vi "SetupApplication.vi"(8 "error in (no error)":errorcluster) -> (0 "error out":errorcluster)   [LabVIEW 2011]
uses:
  080 - TOOLS/Traduction/Dictionnary/EnumCommandDictionnaire.ctl
  050 - CONFIG/00 - ApplicationConfig/Ctrls/EnumFgvConfigCommand.ctl
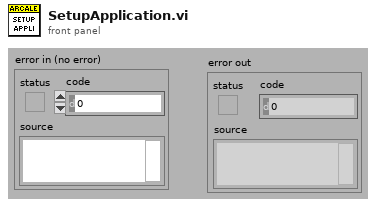
[diagram p1: front panel]
types:
  T1 = typedef "EnumCommandDictionnaire.ctl" = enum16{"Load", "Translate", "Save", "GetDico", "Set : A traduire = Vrai", "Set : A Traduire = Faux", "SetDico"}
  T2 = typedef "EnumFgvConfigCommand.ctl" = enum16{"Load", "Get", "Set", "Save To Disk"}
  T3 = typedef "ApplicationConfig.ctl" = cluster{"Data Path":path, "MessageHandlerConfig":T4, "Simulation":bool, "Dictionnary":string}
  T4 = typedef "MessageHandlerConfig.ctl" = cluster{"Max log files":u32, "Max messages per file":u32}
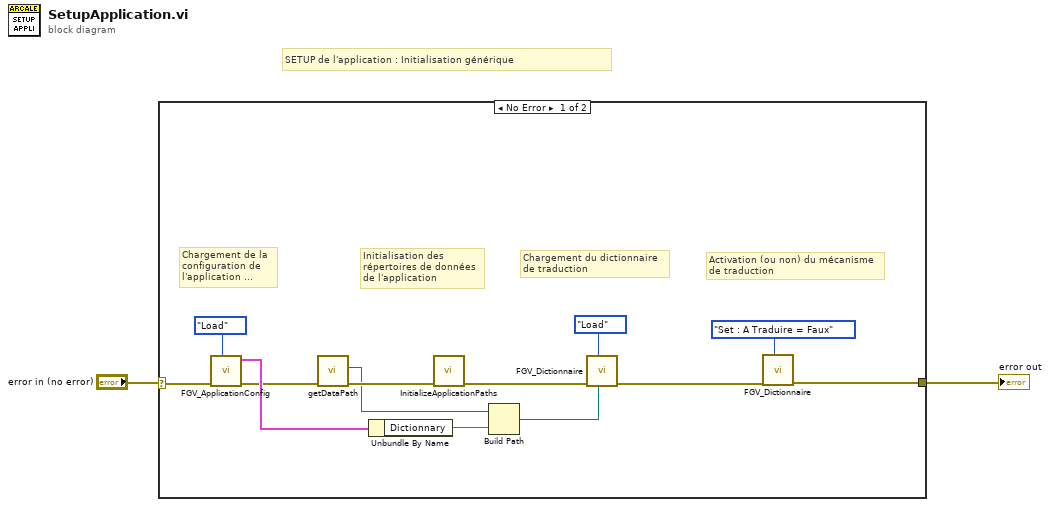
[diagram p0: block diagram]
diagram:
  # "SETUP de l'application : Initialisation générique"
  n1 = case shown="No Error" "error in (no error)" {
    selector: "error in (no error)" -> [w14 w16]
    tunnel: [w9 w16] -> w1
    frame No Error {
      # "Activation (ou non) du mécanisme\nde traduction"
      # "Chargement du dictionnaire\nde traduction"
      # "Initialisation des\nrépertoires de données\nde l'application"
      # "Chargement de la \nconfiguration de \nl'application ..."
      n2 = call "FGV_ApplicationConfig.vi"("Command"=EnumFgvConfigCommand."Load", "error in (no error)"=w14) -> ("error out"=w5:errorcluster, "ApplicationConfigOut"=w8:T3)  [unwired: 8 in]
      n3 = call "getDataPath.vi"("error in (no error)"=w5) -> ("error out"=w4:errorcluster, "DataPath"=w3:path)  [unwired: 9 in]
      n4 = Unbundle By Name(w8) -> ("Dictionnary"=w7:string)
      n5 = call "InitializeApplicationPaths.vi"("error in (no error)"=w4) -> ("error out"=w13:errorcluster)  [unwired: 10 in]
      n6 = Build Path(base path=w3, name or relative path=w7) -> (appended path=w6:path)
      n7 = call "FGV_Dictionnaire.vi"("FichierDictionnaire"=w6, "Command"=EnumCommandDictionnaire."Load", "error in (no error)"=w13) -> ("error out"=w11:errorcluster)  [unwired: 6 in, 2 out]
      n8 = call "FGV_Dictionnaire.vi"("Command"=EnumCommandDictionnaire."Set : A Traduire = Faux", "error in (no error)"=w11) -> ("error out"=w9:errorcluster)  [unwired: 7 in, 2 out]
    }
    frame Error {
    }
  }
  "error out" <- w1
